vi "_Create HTML folders.vi"(0 "HTML File Path":path, 11 "error in (no error)":errorcluster) -> (4 "HTML FIle Path out":path, 6 "HTML Images Folder":path, 8 "HTML Resources Folder":path, 15 "error out":errorcluster)   [LabVIEW 2012]
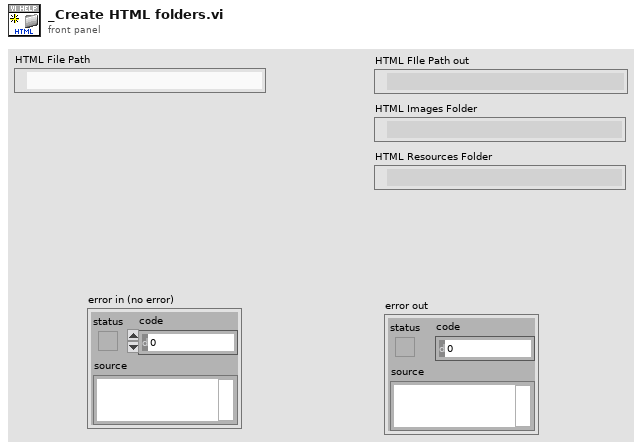
[diagram p1: front panel]
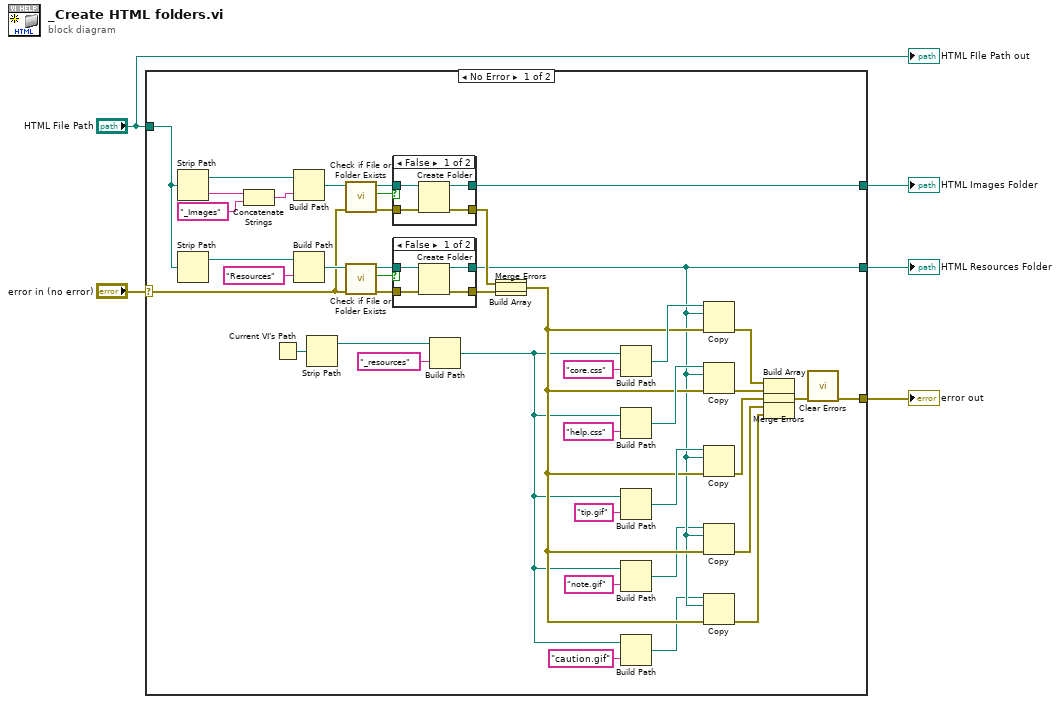
[diagram p0: block diagram]
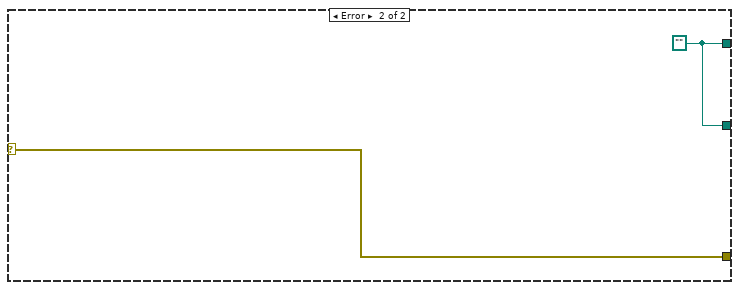
[diagram p4: hidden frame]
diagram:
  n1 = case shown="No Error" "error in (no error)" {
    selector: "error in (no error)" -> [w6 w63]
    tunnel: "HTML File Path" -> [w31 _]
    tunnel: [w22 w62] -> w4
    tunnel: [w21 w63] -> w3
    tunnel: [w15 w62] -> w2
    frame No Error {
      n2 = Strip Path(path=w31) -> (stripped path=w36:path, name=w34:string)
      n3 = Strip Path(path=w31) -> (stripped path=w30:path)  [unwired: 1 out]
      n4 = Concatenate Strings(w34, "_Images" ("name or relative path")) -> (w33:string)
      n5 = Current VI's Path() -> (path=w46:path)
      n6 = Build Path(base path=w36, name or relative path=w33) -> (appended path=w35:path)
      n7 = Build Path(base path=w30, name or relative path="Resources") -> (appended path=w25:path)
      n8 = Strip Path(path=w46) -> (stripped path=w45:path)  [unwired: 1 out]
      n9 = call <vilib>:"Check if File or Folder Exists.vi"("error in (no error)"=w6, "path"=w35) -> ("error out"=w48:errorcluster, "file or folder exists?"=w49:bool, "dup path"=w47:path)  [unwired: 7 in]
      n10 = call <vilib>:"Check if File or Folder Exists.vi"("error in (no error)"=w6, "path"=w25) -> ("error out"=w27:errorcluster, "file or folder exists?"=w28:bool, "dup path"=w26:path)  [unwired: 7 in]
      n11 = case shown="False" w49 {
        tunnel: w47 -> [w59 w61]
        tunnel: w48 -> [w58 w60]
        tunnel: [w57 w61] -> w22
        tunnel: [w56 w60] -> w23
        frame False {
          n12 = Create Folder(path (use dialog)=w59, error in=w58) -> (created path=w57:path, error out=w56:errorcluster)  [unwired: 1 in, 1 out]
        }
        frame True {
        }
      }
      n13 = case shown="False" w28 {
        tunnel: w26 -> [w53 w55]
        tunnel: w27 -> [w52 w54]
        tunnel: [w51 w55] -> w15
        tunnel: [w50 w54] -> w24
        frame False {
          n14 = Create Folder(path (use dialog)=w53, error in=w52) -> (created path=w51:path, error out=w50:errorcluster)  [unwired: 1 in, 1 out]
        }
        frame True {
        }
      }
      n15 = Build Path(base path=w45, name or relative path="_resources") -> (appended path=w9:path)
      n16 = Build Array(w23, w24) -> (w8:errorcluster[])
      n17 = Merge Errors(w8) -> (w16:errorcluster)
      n18 = Build Path(base path=w9, name or relative path="core.css") -> (appended path=w43:path)
      n19 = Build Path(base path=w9, name or relative path="help.css") -> (appended path=w42:path)
      n20 = Build Path(base path=w9, name or relative path="tip.gif") -> (appended path=w17:path)
      n21 = Build Path(base path=w9, name or relative path="note.gif") -> (appended path=w14:path)
      n22 = Build Path(base path=w9, name or relative path="caution.gif") -> (appended path=w13:path)
      n23 = Copy(8:w16, 10:w15, 11:w43) -> (0:w39:errorcluster)  [unwired: 2 in, 2 out]
      n24 = Copy(8:w16, 10:w15, 11:w42) -> (0:w38:errorcluster)  [unwired: 2 in, 2 out]
      n25 = Copy(8:w16, 10:w15, 11:w17) -> (0:w12:errorcluster)  [unwired: 2 in, 2 out]
      n26 = Copy(8:w16, 10:w15, 11:w14) -> (0:w11:errorcluster)  [unwired: 2 in, 2 out]
      n27 = Copy(8:w16, 10:w15, 11:w13) -> (0:w10:errorcluster)  [unwired: 2 in, 2 out]
      n28 = Build Array(w39, w38, w12, w11, w10) -> (w7:errorcluster[])
      n29 = Merge Errors(w7) -> (w37:errorcluster)
      n30 = call <vilib>:"Clear Errors.vi"("error in (no error)"=w37) -> ("error out"=w21:errorcluster)  [unwired: 6 in]
    }
    frame Error {
      w62 = path ""
    }
  }
  "error out" <- w3
  "HTML Images Folder" <- w4
  "HTML Resources Folder" <- w2
  "HTML FIle Path out" <- "HTML File Path"
